vi "FGV_BenchConfig.vi"(7 "Command":T2, 8 "error in (no error)":errorcluster, 11 "BenchConfigIn":T1) -> (0 "error out":errorcluster, 3 "BenchConfigOut":T1)   [LabVIEW 2011]
uses:
  00 - ApplicationConfig/Ctrls/EnumFgvConfigCommand.ctl
  BenchConfig.ctl
panel:
  # "A configurer"
  # "A configurer"
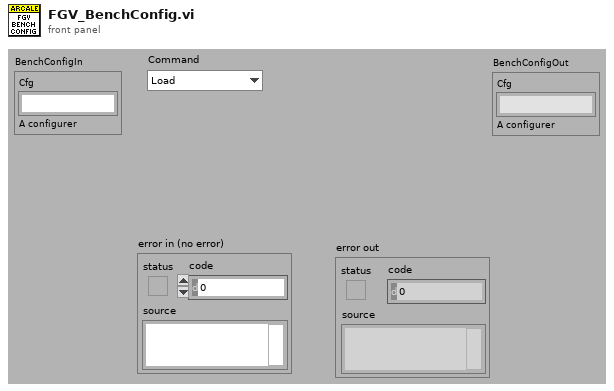
[diagram p1: front panel]
types:
  T1 = typedef "BenchConfig.ctl" = cluster{"Cfg":string}
  T2 = typedef "EnumFgvConfigCommand.ctl" = enum16{"Load", "Get", "Set", "Save To Disk"}
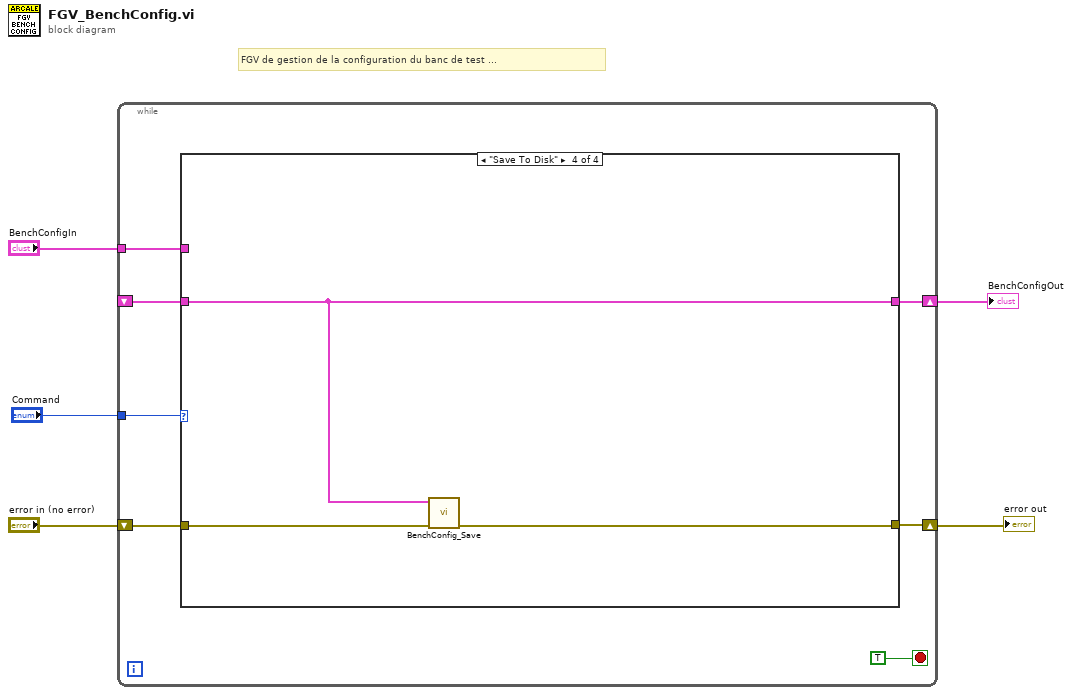
[diagram p0: block diagram]
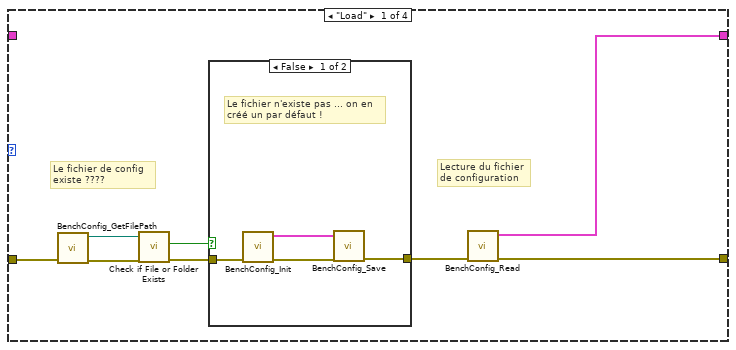
[diagram p2: hidden frame]
diagram:
  # "FGV de gestion de la configuration du banc de test ..."
  n1 = while {
    shift-right: [w9] -> w4
    shift-left: "error in (no error)" -> [w10]
    tunnel: "Command" -> [w11]
    shift-right: [w8] -> w2
    shift-left: _ -> [w7]
    tunnel: "BenchConfigIn" -> [w6]
    stop <- TRUE stop-if-true
    n2 = case shown="\"Save To Disk\"" w11 {
      tunnel: w10 -> [w20 w26 w28 w32]
      tunnel: [w14 w26 w28 w31] -> w9
      tunnel: [w13 w27 w29 w30] -> w8
      tunnel: w7 -> [_ w27 _ w30]
      tunnel: w6 -> [_ _ w29 _]
      frame "Load" {
        # "Lecture du fichier\nde configuration"
        # "Le fichier de config \nexiste ????"
        n3 = call "BenchConfig_GetFilePath.vi"("error in (no error)"=w20) -> ("error out"=w19:errorcluster, "BenchConfigFilePath"=w18:path)  [unwired: 9 in]
        n4 = call <vilib>:"Check if File or Folder Exists.vi"("error in (no error)"=w19, "path"=w18) -> ("error out"=w16:errorcluster, "file or folder exists?"=w17:bool)  [unwired: 7 in, 1 out]
        n5 = case shown="False" w17 {
          tunnel: w16 -> [w24 w25]
          tunnel: [w21 w25] -> w15
          frame False {
            # "Le fichier n'existe pas ... on en \ncréé un par défaut !"
            n6 = call "BenchConfig_Init.vi"("error in (no error)"=w24) -> ("error out"=w23:errorcluster, "BenchConfig"=w22:T1)  [unwired: 9 in]
            n7 = call "BenchConfig_Save.vi"("error in (no error)"=w23, "BenchConfig"=w22) -> ("error out"=w21:errorcluster)  [unwired: 9 in]
          }
          frame True {
            # "Le fichier existe ...."
          }
        }
        n8 = call "BenchConfig_Read.vi"("error in (no error)"=w15) -> ("error out"=w14:errorcluster, "BenchConfig"=w13:T1)  [unwired: 9 in]
      }
      frame "Get" {
      }
      frame "Set" {
      }
      frame "Save To Disk" {
        n9 = call "BenchConfig_Save.vi"("error in (no error)"=w32, "BenchConfig"=w30) -> ("error out"=w31:errorcluster)  [unwired: 9 in]
      }
    }
  }
  "error out" <- w4
  "BenchConfigOut" <- w2
